vi "Scalar Get Info.vi"(8 "error in (no error)":errorcluster, 11 "Scalar DVR in":refnum<data-value>) -> (0 "error out":errorcluster, 3 "Scalar DVR out":refnum<data-value>)   [LabVIEW 2012, in "MDSplus.lvlib"]
uses:
  <vilib>/MDSplus/Library/MDSplus.lvlib
  <vilib>/MDSplus/Classes/Data_Class/Scalar_Class/Scalar.lvclass
panel:
  out "Dimensions out":i32[](array[numeric])
  out "Data length out":i16
  out "Data type out":u8
  out "Class type out":u8
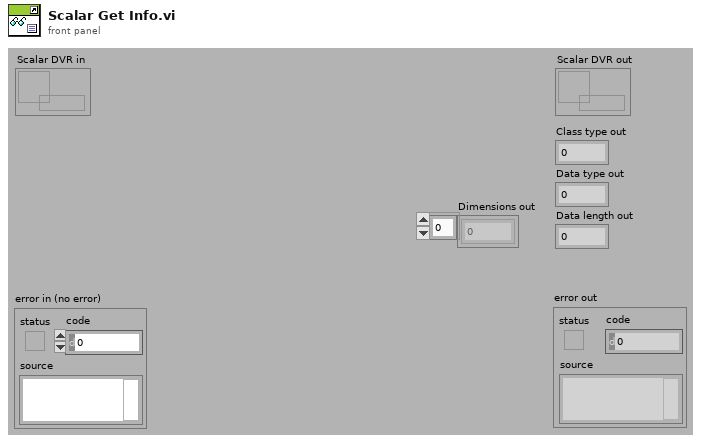
[diagram p1: front panel]
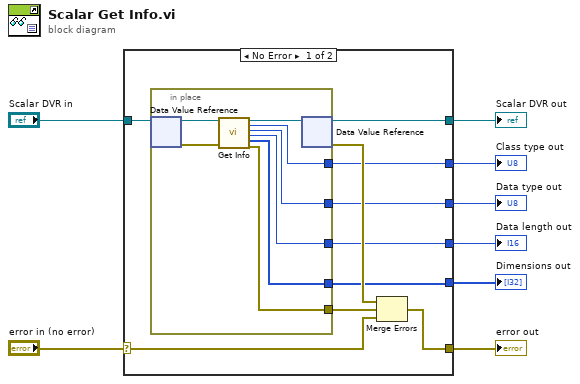
[diagram p0: block diagram]
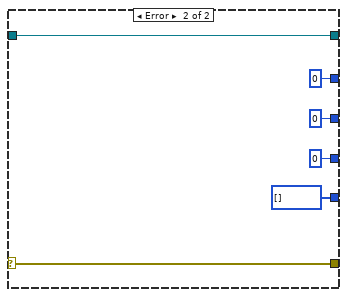
[diagram p2: hidden frame]
diagram:
  n1 = case shown="No Error" "error in (no error)" {
    selector: "error in (no error)" -> [w16 w32]
    tunnel: "Scalar DVR in" -> [w18 w31]
    tunnel: [w14 w32] -> w8
    tunnel: [w13 w31] -> w5
    tunnel: [w12 u8 0 ("Class type out")] -> w4
    tunnel: [w11 u8 0 ("Data type out")] -> w3
    tunnel: [w10 i16 0 ("Data length out")] -> w2
    tunnel: [w9 i32[] [] ("Dimensions out")] -> w1
    frame No Error {
      n2 = in-place {
        in-place-border: [w24] -> w17
        in-place-border: [w22] -> w12
        in-place-border: [w21] -> w11
        in-place-border: [w20] -> w10
        in-place-border: [w19] -> w9
        n3 = in-place-dvr #1(w18) -> (w26:refnum<class "Scalar.lvclass">, w23:errorcluster)
        n4 = call-dynamic "Get Info.vi"("Scalar in"=w26, "error in (no error)"=w23) -> ("Scalar out"=w25:refnum<class "Scalar.lvclass">, "Class type out"=w22:u8, "Data type out"=w21:u8, "Data length out"=w20:i16, "Dimensions out"=w19:i32[], "error out"=w24:errorcluster)  [unwired: 12 in]
        n5 = in-place-dvr #1(w25) -> (w13:refnum<data-value>, w15:errorcluster)
      }
      n6 = Merge Errors(w15, w17, w16) -> (w14:errorcluster)
    }
    frame Error {
    }
  }
  "error out" <- w8
  "Scalar DVR out" <- w5
  "Class type out" <- w4
  "Data type out" <- w3
  "Data length out" <- w2
  "Dimensions out" <- w1
